vi "set_config_cluster.vi"(8 "error in (no error)":errorcluster, 10 "config cluster variant":variant, 11 "GenericObjective in":refnum<class "GenericObjective.lvclass">) -> (0 "error out":errorcluster, 3 "GenericObjective out":refnum<class "GenericObjective.lvclass">)   [LabVIEW 2010, in "GenericObjective.lvclass"]
uses:
  GenericObjective.lvclass
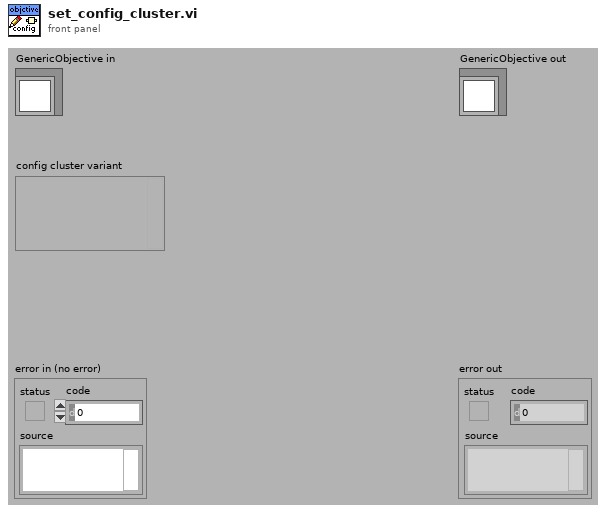
[diagram p1: front panel]
types:
  T1 = typedef "GenericObjective.lvclass/config_data_cluster.ctl" = cluster{"magnification":dbl}
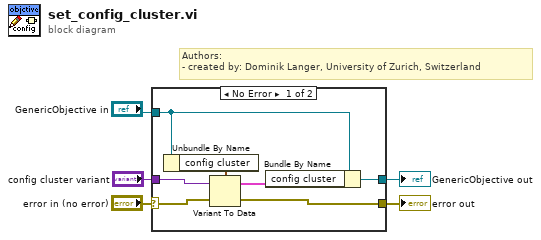
[diagram p0: block diagram]
diagram:
  # "Authors: \n- created by: Dominik Langer, University of Zurich, Switzerland"
  n1 = case shown="No Error" "error in (no error)" {
    selector: "error in (no error)" -> [w10 w14]
    tunnel: "config cluster variant" -> [w9 _]
    tunnel: "GenericObjective in" -> [w8 w13]
    tunnel: [w7 w14] -> w2
    tunnel: [w6 w13] -> w1
    frame No Error {
      n2 = Unbundle By Name(w8) -> ("config cluster"=w11:T1)
      n3 = Variant To Data(error in=w10, Variant=w9, type=w11) -> (error out=w7:errorcluster, data=w12:cluster{})
      n4 = Bundle By Name(cluster=w8, "config cluster"=w12) -> (w6:refnum<class "GenericObjective.lvclass">)
    }
    frame Error {
    }
  }
  "error out" <- w2
  "GenericObjective out" <- w1
